vi "Com_Panel_Panel Open.vi"(8 "error in":errorcluster, 10 "Activate?":bool=TRUE, 11 "VI Refnum In":refnum<vi>) -> (0 "error out":errorcluster, 3 "VI Refnum Out":refnum<vi>)   [LabVIEW 2016]
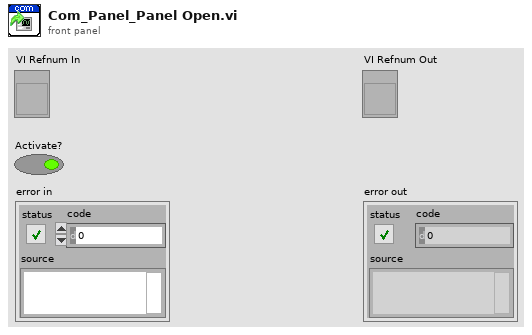
[diagram p1: front panel]
types:
  T1 = enum32{"Invalid", "Standard", "Closed", "Hidden", "Minimized", "Maximized"}
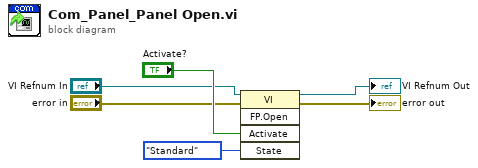
[diagram p0: block diagram]
diagram:
  n1 = invoke class="VI" method="FP.Open"(reference="VI Refnum In", error in="error in", "Activate"="Activate?", "State"=T1."Standard") -> (reference out=→"VI Refnum Out":refnum<vi>, error out=→"error out":errorcluster)  [unwired: 1 in, 3 out]
